vi "streak calculations.vi"(8 "error in (no error)":errorcluster, 10 "Streak":T1 {"streak step" min=-1.0 max=1.0; "streak length" min=-1.0 max=1.0}, 11 "curve data":cluster{"X":dbl[], "Y ":dbl[]}) -> (0 "error out":errorcluster, 2 "Streak out":T1 {"streak step" min=-1.0 max=1.0; "streak length" min=-1.0 max=1.0}, 3 "data for graph":cluster{"X":dbl[], "Y":dbl[]})   [LabVIEW 2020]
uses:
  controls/streak settings.ctl
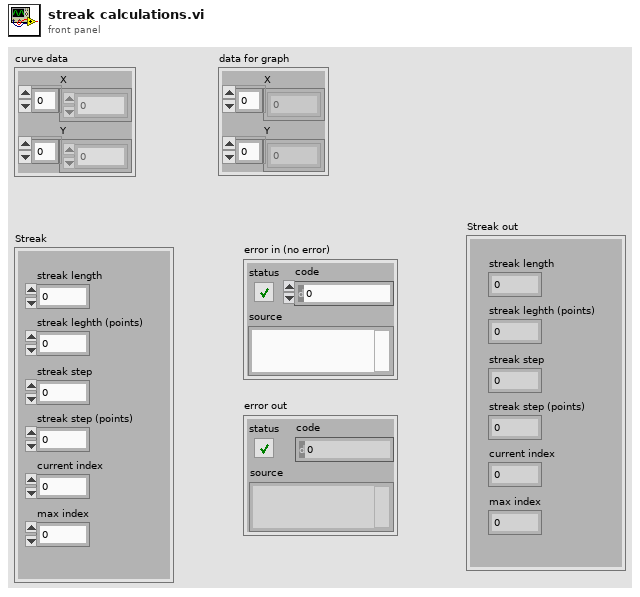
[diagram p1: front panel]
types:
  T1 = typedef "streak settings.ctl" = cluster{"streak length":dbl, "streak leghth (points)":i32, "streak step":dbl, "streak step (points)":i32, "current index":i32, "max index":i32}
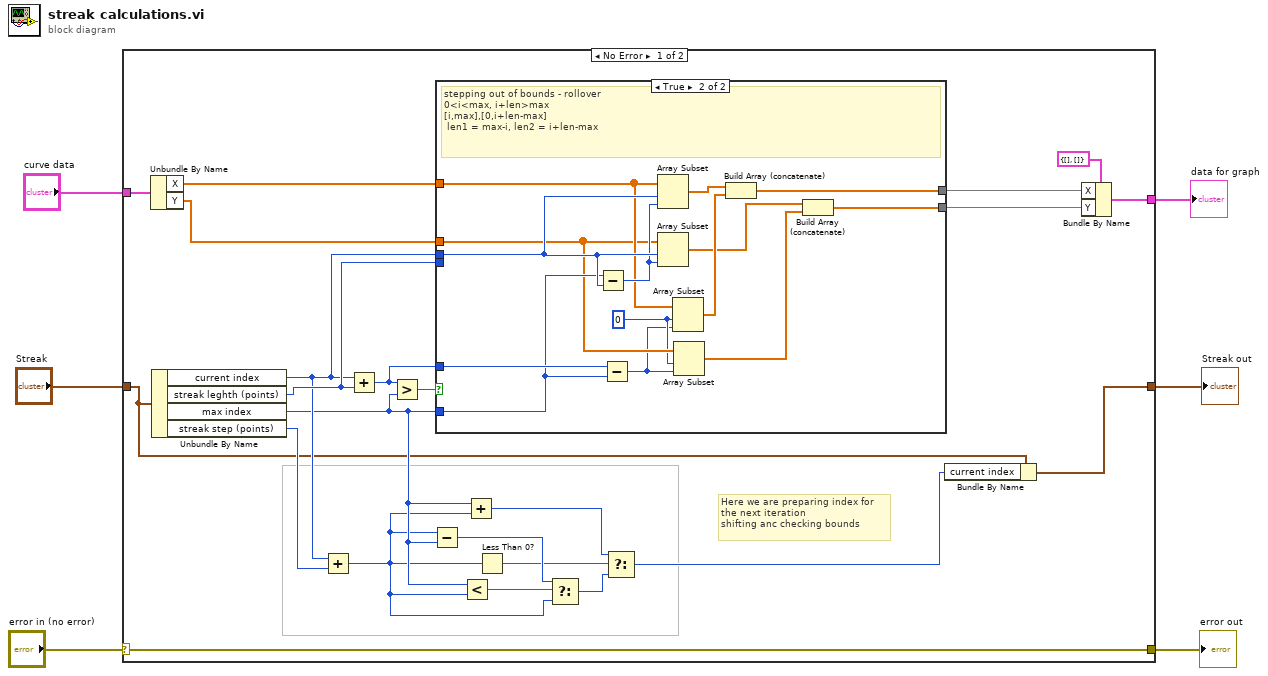
[diagram p0: block diagram]
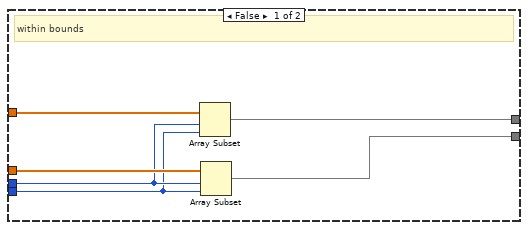
[diagram p2: hidden frame]
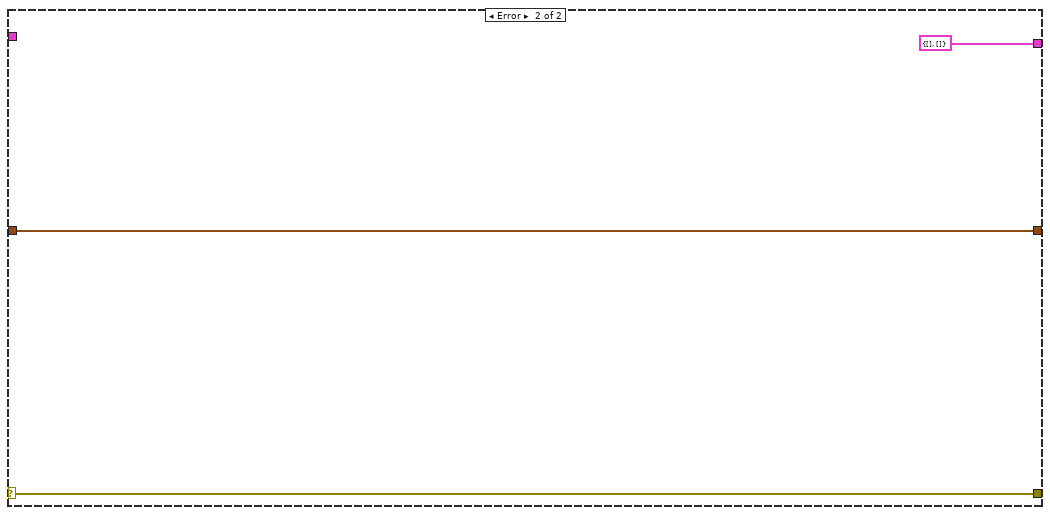
[diagram p3: hidden frame]
diagram:
  n1 = case shown="No Error" "error in (no error)" {
    selector: "error in (no error)" -> [w19 w52]
    tunnel: [w19 w52] -> w5
    tunnel: [w28 cluster{"X":dbl[], "Y":dbl[]} {"X"=[], "Y"=[]}] -> w4
    tunnel: "Streak" -> [w9 w50]
    tunnel: "curve data" -> [w27 _]
    tunnel: [w8 w50] -> w1
    frame No Error {
      # "Here we are preparing index for \nthe next iteration\nshifting anc checking bounds"
      n2 = Unbundle By Name(w27) -> ("X"=w25:dbl[], "Y"=w24:dbl[])
      n3 = Unbundle By Name(w9) -> ("current index"=w18:i32, "streak leghth (points)"=w26:i32, "max index"=w12:i32, "streak step (points)"=w17:i32)
      n4 = Add(x=w18, y=w17) -> (x+y=w11:i32)
      n5 = Add(x=w18, y=w26) -> (x+y=w20:i32)
      n6 = Greater?(x=w20, y=w12) -> (0:w21:bool)
      n7 = Subtract(x=w11, y=w12) -> (x-y=w15:i32)
      n8 = case shown="True" w21 {
        tunnel: w25 -> [w35 w45]
        tunnel: w24 -> [w34 w44]
        tunnel: [w33 w39] -> w23
        tunnel: [w32 w38] -> w22
        tunnel: w18 -> [w31 w49]
        tunnel: w26 -> [w30 _]
        tunnel: w12 -> [_ w46]
        tunnel: w20 -> [_ w47]
        frame False {
          # "within bounds"
          n9 = Array Subset(array=w35, index=w31, length=w30) -> (w33:dbl[])
          n10 = Array Subset(array=w34, index=w31, length=w30) -> (w32:dbl[])
        }
        frame True {
          w43 = 0 ("index")
          # "stepping out of bounds - rollover\n0<i<max, i+len>max\n[i,max],[0,i+len-max]\n len1 = max-i, len2 = i+len-max"
          n11 = Subtract(x=w46, y=w49) -> (x-y=w48:i32)
          n12 = Subtract(x=w47, y=w46) -> (x-y=w42:i32)
          n13 = Array Subset(array=w45, index=w49, length=w48) -> (w41:dbl[])
          n14 = Array Subset(array=w44, index=w49, length=w48) -> (w37:dbl[])
          n15 = Array Subset(array=w45, index=w43, length=w42) -> (w40:dbl[])
          n16 = Array Subset(array=w44, index=w43, length=w42) -> (w36:dbl[])
          n17 = Build Array (concatenate)(w41, w40) -> (w39:dbl[])
          n18 = Build Array (concatenate)(w37, w36) -> (w38:dbl[])
        }
      }
      n19 = Less?(x=w12, y=w11) -> (x < y?=w16:bool)
      n20 = Add(x=w12, y=w11) -> (x+y=w10:i32)
      n21 = Less Than 0?(x=w11) -> (x < 0?=w14:bool)
      n22 = Select(t=w15, s=w16, f=w11) -> (s? t:f=w13:i32)
      n23 = Select(t=w10, s=w14, f=w13) -> (s? t:f=w7:i32)
      n24 = Bundle By Name(cluster=w9, "current index"=w7) -> (w8:T1)
      n25 = Bundle By Name(cluster=cluster{"X":dbl[], "Y":dbl[]} {"X"=[], "Y"=[]}, "X"=w23, "Y"=w22) -> (w28:cluster{"X":dbl[], "Y":dbl[]})
    }
    frame Error {
    }
  }
  "data for graph" <- w4
  "error out" <- w5
  "Streak out" <- w1
